vi "Waveform Peak Detection.vi"   [LabVIEW 2020, in "NI_MAPro.lvlib"]
doc: "Finds the locations, amplitudes, and second derivatives of peaks and valleys in <B>Signal In</B>. Wire data to the <B>Signal In</B> input to determine the polymorphic instance to use or manually select the instance."
uses:
  NI_MAPro.lvlib
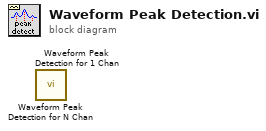
[diagram p0: block diagram]
diagram:
  n1 = call "Waveform Peak Detection for N Chan.vi"() -> ()  [unwired: 7 in, 5 out]
  n2 = call "Waveform Peak Detection for 1 Chan.vi"() -> ()  [unwired: 7 in, 5 out]
